vi "bats.parser.test.Time.Twice.vi"(10 "Expected OrderBook.Command[]":T1[](array[typedef])=[{"OrderBook Command.Type"=enum."Time", "Side (U8)"=0, "Order Id (U64)"=0, "Quantity (U32)"=0, "Symbol (U64)"=0, "Price (U64)"=0, "Executed Quantity (U32)"=0, "Cancelled Quantity (U32)"=0, "Seconds (U64)"=447000, "Nanoseconds (U64)"=0}, {"OrderBook Command.Type"=enum."Time", "Side (U8)"=0, "Order Id (U64)"=0, "Quantity (U32)"=0, "Symbol (U64)"=0, "Price (U64)"=0, "Executed Quantity (U32)"=0, "Cancelled Quantity (U32)"=0, "Seconds (U64)"=448000, "Nanoseconds (U64)"=0}] {"Side (U8)" format="%.0x"; "Order Id (U64)" format="%.0x"; "Symbol (U64)" format="%.0x"}, 11 "Test.Messages":T3[](array[typedef])=[{"MessageType"=enum."Time", "AddOrderLong.Parms"={"Time Offset"=447000, "Order Id"="ORID0001", "Side Indicator"="B", "Quantity"=20000, "Symbol"="AAPL", "Price"=0.905, "Add Flags"=1}, "Time.Parms"={"Seconds Since Midnight"=447000}, "SequencedUnitHeader.Parms"={"Hdr Count"=32, "Hdr Unit"=1, "Hdr Sequence"=1, "Starting Sequence"=1}}, {"MessageType"=enum."Time", "AddOrderLong.Parms"={"Time Offset"=447000, "Order Id"="ORID0001", "Side Indicator"="B", "Quantity"=20000, "Symbol"="AAPL", "Price"=0.905, "Add Flags"=1}, "Time.Parms"={"Seconds Since Midnight"=448000}, "SequencedUnitHeader.Parms"={"Hdr Count"=32, "Hdr Unit"=1, "Hdr Sequence"=1, "Starting Sequence"=1}}]) -> ()   [LabVIEW 2022 SP3]
uses:
  Message.Spec.ctl
  pitch/MessageType.ctl
  pitch/AddOrderLong/AddOrderLong.Parameters.ctl
  pitch/Time/Time.Parameters.ctl
  pitch/SequencedUnitHeader/SequencedUnitHeader.Parameters.ctl
  arty/orderbook/orderbook.command.ctl
  arty/orderbook/orderbook.command.type.ctl
  pitch/Time/Time.lvclass
  pitch/AddOrderLong/AddOrderLong.lvclass
  pitch/SequencedUnitHeader/SequencedUnitHeader.lvclass
panel:
  out "Passed":bool
  out "OrderBook.Command[]":T1[](array[typedef]) {"Side (U8)" format="%.0x"; "Order Id (U64)" format="%.0x"; "Symbol (U64)" format="%.0x"}
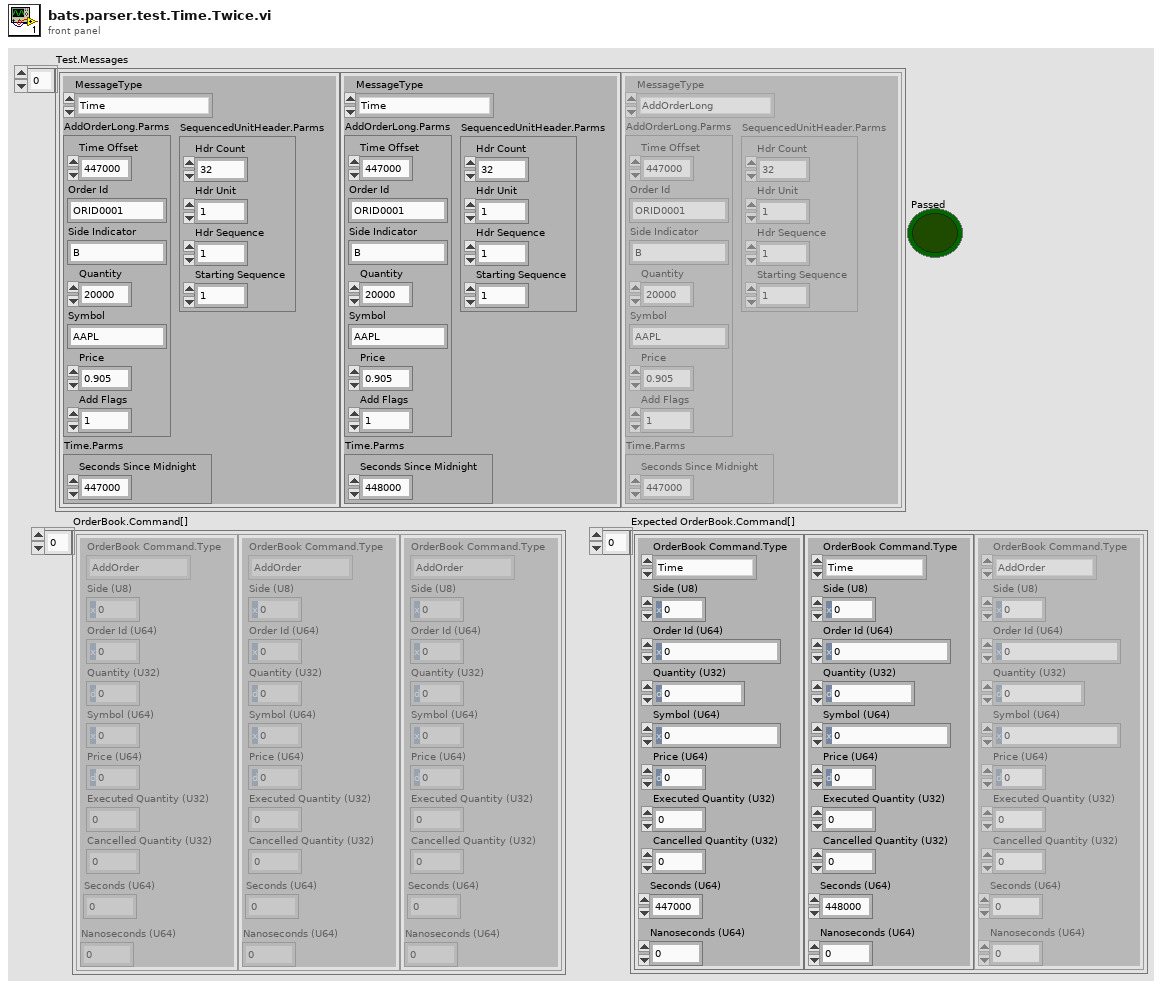
[diagram p1: front panel]
types:
  T1 = typedef "orderbook.command.ctl" = cluster{"OrderBook Command.Type":T2, "Side (U8)":u8, "Order Id (U64)":u64, "Quantity (U32)":u32, "Symbol (U64)":u64, "Price (U64)":u64, "Executed Quantity (U32)":u32, "Cancelled Quantity (U32)":u32, "Seconds (U64)":u64, "Nanoseconds (U64)":u64}
  T2 = typedef "orderbook.command.type.ctl" = enum16{"Time", "AddOrder", "OrderExecuted", "ReduceSize", "ModifyOrder", "DeleteOrder", "Get.All.Orders", "Get.Top"}
  T3 = typedef "Message.Spec.ctl" = cluster{"MessageType":T4, "AddOrderLong.Parms":T5, "Time.Parms":T6, "SequencedUnitHeader.Parms":T7}
  T4 = typedef "MessageType.ctl" = enum16{"SequencedUnitHeader", "AddOrderLong", "AddOrderShort", "AddOrderExpanded", "Time"}
  T5 = typedef "AddOrderLong.lvclass/AddOrderLong.Parameters.ctl" = cluster{"Time Offset":u32, "Order Id":string, "Side Indicator":string, "Quantity":u32, "Symbol":string, "Price":dbl, "Add Flags":u8}
  T6 = typedef "Time.lvclass/Time.Parameters.ctl" = cluster{"Seconds Since Midnight":u32}
  T7 = typedef "SequencedUnitHeader.lvclass/SequencedUnitHeader.Parameters.ctl" = cluster{"Hdr Count":u8, "Hdr Unit":u8, "Hdr Sequence":u32, "Starting Sequence":u32}
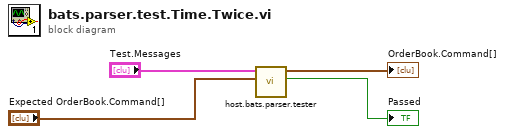
[diagram p0: block diagram]
diagram:
  n1 = call "host.bats.parser.tester.vi"("Expected OrderBook.Command[]"="Expected OrderBook.Command[]", "Test.Messages"="Test.Messages") -> ("Passed"=→"Passed":bool, "OrderBook.Command[]"=→"OrderBook.Command[]":T1[])  [unwired: 5 in, 3 out]
